vi "Generate Correlated Signal.vi"() -> ()   [LabVIEW 2023]
doc: "This VI demonstrates how to generate 3 correlated signals and display correlation using a scatter plot. \n\nIt also demonstrates how to convert from Correlation Matrix to Covariance Matrix."
uses:
  <vilib>/Analysis/_algsub.llb/Matrix Type for Test.ctl
  <vilib>/Analysis/7linalg.llb/Eigenvalue and Vectors Output Option.ctl
  <vilib>/Analysis/baseanly.llb/Real A x B.vi
  <vilib>/Analysis/baseanly.llb/Complex A x B.vi
  <vilib>/Analysis/7linalg.llb/Create Special Real Matrix.vi
  <vilib>/Analysis/_algsub.llb/Test Real Matrix Type.vi
  <vilib>/Utility/error.llb/Error Cluster From Error Code.vi
  <vilib>/Analysis/7linalg.llb/Real Eigenvalues and Vectors.vi
  <vilib>/Analysis/7linalg.llb/Create Special Complex Matrix.vi
  <vilib>/Analysis/Matrix/Numeric/Complex/Complex To Cartesian - CM.vi
  <vilib>/Analysis/BLAS.llb/dgemv - General Matrix-Vector Product (DBL).vi
  <vilib>/ErrorRing/Error Ring.xnode
  <vilib>/Analysis/NI_AALPro.lvlib
  <vilib>/Analysis/NI_AALBase.lvlib
  <vilib>/gmath/NI_Gmath.lvlib
  <vilib>/Analysis/Matrix/NI_Matrix.lvlib
  <vilib>/Analysis/NI_AALBLAS.lvlib
panel:
  in  "Description":string="Overview: This VI demonstrates how to generate 3 correlated signals and display correlation using a scatter plot. It also demonstrates how to convert from Correlation Matrix to Covariance Matrix.\nRequirements: LabVIEW Full Development System\nInstructions: \n1. Enter the Expected Values, Correlation Matrix, and Standard Deviation of the three signals. \n2. Run the VI and verify the calculated Covariance Matrix and the scatter plot matrix. Notice that, depending on the values entered, if the resulting Covariance Matrix is not Positive Semi-definite, an error will be generated. "
  in  "Tab Control":enum32{"Scatter Plot Matrix", "Time signal"}(tab)
  out "X2 vs X1 5":cluster{"Data Set 1":dbl[], "Data Set 2":dbl[]}(graph)
  out "X3 vs X1":cluster{"Data Set 1":dbl[], "Data Set 2":dbl[]}(graph)
  out "X3 vs X2":cluster{"Data Set 1":dbl[], "Data Set 2":dbl[]}(graph)
  out "X1 vs X2":cluster{"Data Set 1":dbl[], "Data Set 2":dbl[]}(graph)
  out "X1 vs X3":cluster{"Data Set 1":dbl[], "Data Set 2":dbl[]}(graph)
  out "X2 vs X3":cluster{"Data Set 1":dbl[], "Data Set 2":dbl[]}(graph)
  out "Variable 3":dbl[](graph)
  out "Variable 2":dbl[](graph)
  out "Variable 1":dbl[](graph)
  in  "Standard Deviation":dbl[](array[numeric])=[2.0, 1.0, 4.0]
  in  "number of points":i32=1000
  out "Covariance Matrix":dbl[][](array[numeric]) format="%#.4g"
  out "mean vector":dbl[](array[numeric]) format="%#.4g"
  in  "Expected Values":dbl[](array[numeric])=[100.0, 1.0, 10.0]
  in  "Correlation Matrix":dbl[][](array[numeric])=[[1.0, 0.9, 0.0], [0.9, 1.0, -0.4], [0.0, -0.4, 1.0]]
  in  "seed":i32=2
  # "Input Statistics to generate"
  # "Measure Statistics"
  # "Variable 1"
  # "Variable 2"
  # "Variable 3"
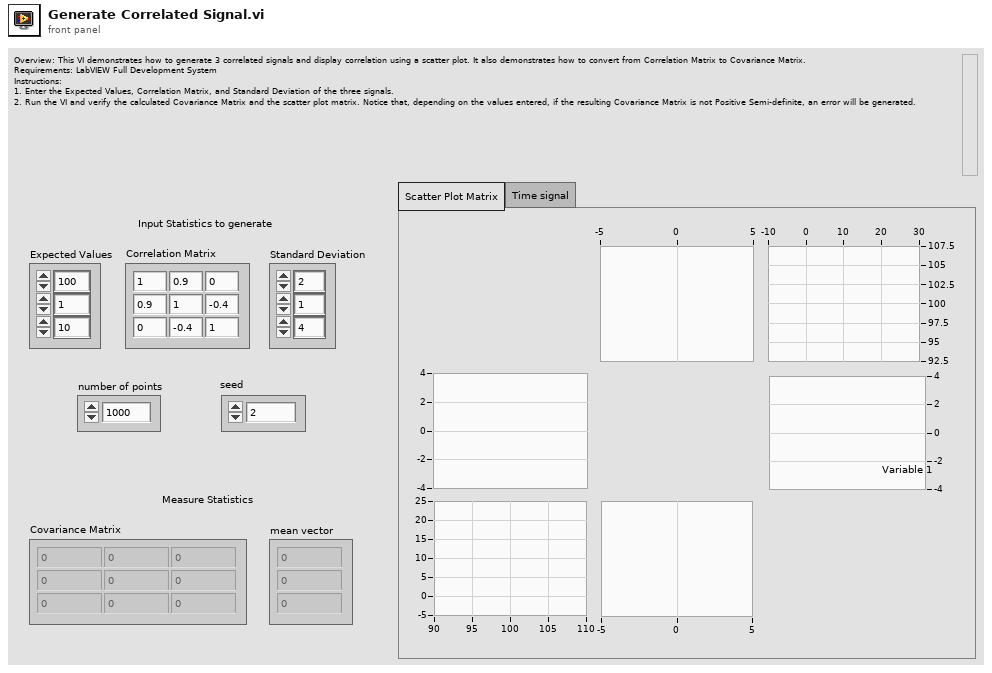
[diagram p1: front panel]
types:
  T1 = typedef "NI_AALPro.lvlib/Matrix Type for Test.ctl" = i32
  T2 = typedef "NI_Matrix.lvlib/RealMatrix.ctl" = dbl[][]
  T3 = typedef "NI_AALPro.lvlib/Eigenvalue and Vectors Output Option.ctl" = i32
  T4 = typedef "NI_Matrix.lvlib/ComplexMatrix.ctl" = cdb[][]
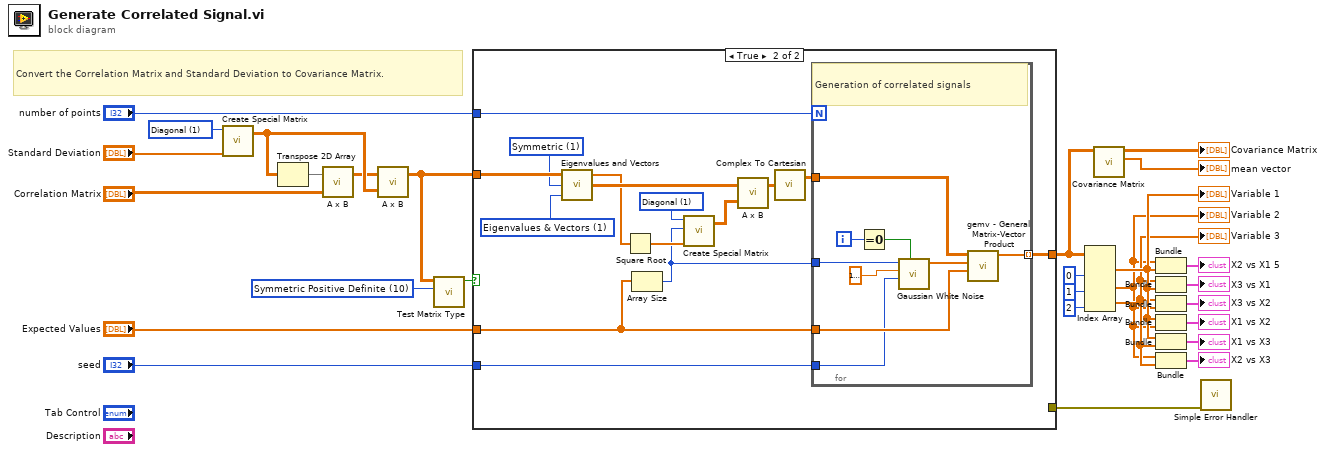
[diagram p0: block diagram]
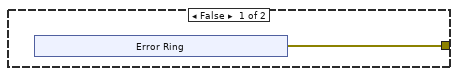
[diagram p2: hidden frame]
diagram:
  w15 = 1 items=["Identity", "Diagonal", "Toeplitz", "Vandermonde", "Companion", "Hankel", "Hadamard", "Wilkinson", "Hilbert", "Inverse Hilbert", "Rosser", "Pascal"] ("matrix type")
  w25 = T1 10 items=["Symmetric Positive Definite"=10, "Symmetric Positive Semi-Definite"=11, "Symmetric"=20, "Hermitian"=21] ("matrix type")
  # "Convert the Correlation Matrix and Standard Deviation to Covariance Matrix."
  n1 = call-poly <vilib>:"Create Special Matrix.vi"("matrix type"=w15, "Input Vector1"="Standard Deviation") -> ("Special Matrix"=w10:T2)  [unwired: 3 in, 1 out]
  n2 = Transpose 2D Array(2D array=w10) -> (transposed array=w13:T2)
  n3 = call-poly <vilib>:"A x B.vi"("B"="Correlation Matrix", "A"=w13) -> ("A x B"=w9:T2)  [unwired: 1 out]
  n4 = call-poly <vilib>:"A x B.vi"("B"=w10, "A"=w9) -> ("A x B"=w14:T2)  [unwired: 1 out]
  n5 = call-poly <vilib>:"Test Matrix Type.vi"("matrix type"=w25, "Input Matrix"=w14) -> ("is type?"=w8:bool)  [unwired: 8 in, 1 out]
  n6 = case shown="True" w8 {
    tunnel: w14 -> [_ w45]
    tunnel: [w29 _] -> w7
    tunnel: [_ w41] -> w21
    tunnel: "Expected Values" -> [_ w40]
    tunnel: "seed" -> [_ w39]
    tunnel: "number of points" -> [_ w38]
    frame False {
      n7 = xnode "Error Ring"() -> ("error out"=w29:errorcluster)
    }
    frame True {
      w35 = 1 items=["Identity", "Diagonal", "Toeplitz", "Vandermonde", "Companion", "Hankel", "Hadamard", "Wilkinson", "Hilbert", "Inverse Hilbert", "Rosser", "Pascal"] ("matrix type")
      w36 = T3 1 items=["Eigenvalues", "Eigenvalues & Vectors"] ("output option")
      w37 = 1 items=["General", "Symmetric"] ("matrix type")
      n8 = call-poly <vilib>:"Eigenvalues and Vectors.vi"("output option"=w36, "matrix type"=w37, "Input Matrix"=w45) -> ("Eigenvectors"=w48:T4, "Eigenvalues"=w47:cdb[])  [unwired: 1 out]
      n9 = Square Root(x=w47) -> (sqrt(x)=w46:cdb[])
      n10 = Array Size(array=w40) -> (size(s)=w42:i32)
      n11 = call-poly <vilib>:"Create Special Matrix.vi"("matrix type"=w35, "matrix size"=w42, "Input Vector1"=w46) -> ("Special Matrix"=w49:T4)  [unwired: 1 in, 2 out]
      n12 = call-poly <vilib>:"A x B.vi"("B"=w49, "A"=w48) -> ("A x B"=w44:T4)  [unwired: 1 out]
      n13 = call-poly <vilib>:"Complex To Cartesian.vi"("Complex Matrix R + Ii"=w44) -> ("Real Matrix R"=w43:T2)  [unwired: 1 out]
      n14 = for {
        N: w38 -> [_]
        tunnel: w43 -> [w55]
        tunnel: w40 -> [w53]
        tunnel: w42 -> [w56]
        tunnel: [w52] -> w41 mode=indexing
        tunnel: w39 -> [w51]
        i -> [w58]
        # "Generation of correlated signals"
        n15 = Equal To 0?(x=w58) -> (x = 0?=w57:bool)
        n16 = call <vilib>:"Gaussian White Noise.vi"("initialize?"=w57, "seed"=w51, "standard deviation"=1.0000000000000002, "samples"=w56) -> ("Gaussian noise pattern"=w54:dbl[])  [unwired: 6 in, 1 out]
        n17 = call-poly <vilib>:"gemv - General Matrix-Vector Product.vi"("y"=w53, "x"=w54, "A"=w55) -> ("dgemv"=w52:dbl[])  [unwired: 7 in, 1 out]
      }
    }
  }
  n18 = Index Array(array=w21, index (col) #1=0 ("disabled index (col)"), index (col) #2=1 ("index (col)"), index (col) #3=2 ("index (col)")) -> (element #1=w3:dbl[], element #2=w1:dbl[], element #3=w2:dbl[])  [unwired: 3 in]
  "Variable 1" <- w3
  "Variable 2" <- w1
  "Variable 3" <- w2
  n19 = call <vilib>:"Covariance Matrix.vi"("X"=w21) -> ("mean vector"=→"mean vector":dbl[], "covariance matrix V"=→"Covariance Matrix":T2)  [unwired: 9 in]
  n20 = Bundle("dgemv"=w1, "dgemv"=w3) -> (→"X2 vs X1 5":cluster{"dgemv":dbl[], "dgemv":dbl[]})  [unwired: 1 in]
  n21 = Bundle("dgemv"=w2, "dgemv"=w3) -> (→"X3 vs X1":cluster{"dgemv":dbl[], "dgemv":dbl[]})  [unwired: 1 in]
  n22 = Bundle("dgemv"=w2, "dgemv"=w1) -> (→"X3 vs X2":cluster{"dgemv":dbl[], "dgemv":dbl[]})  [unwired: 1 in]
  n23 = Bundle("dgemv"=w3, "dgemv"=w1) -> (→"X1 vs X2":cluster{"dgemv":dbl[], "dgemv":dbl[]})  [unwired: 1 in]
  n24 = Bundle("dgemv"=w3, "dgemv"=w2) -> (→"X1 vs X3":cluster{"dgemv":dbl[], "dgemv":dbl[]})  [unwired: 1 in]
  n25 = Bundle("dgemv"=w1, "dgemv"=w2) -> (→"X2 vs X3":cluster{"dgemv":dbl[], "dgemv":dbl[]})  [unwired: 1 in]
  n26 = call <vilib>:"Simple Error Handler.vi"("error in (no error)"=w7) -> ()  [unwired: 4 in, 5 out]
